vi "U8 Array Reverse Bit Order.vi"(1 "U8 Array Data In":u8[](array[numeric]) format="%02x") -> (0 "U8 Array Data Out":u8[](array[numeric]) format="%02x")   [LabVIEW 2016, in "SPIVI.lvlib"]
uses:
  SPIVI.lvlib
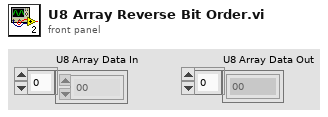
[diagram p1: front panel]
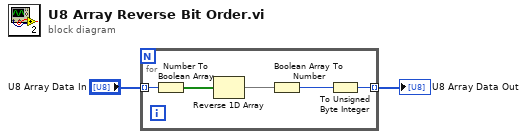
[diagram p0: block diagram]
diagram:
  n1 = for {
    tunnel: "U8 Array Data In" -> [w4] mode=indexing
    tunnel: [w3] -> w1 mode=indexing
    n2 = Number To Boolean Array(number=w4) -> (Boolean array=w7:bool[])
    n3 = Reverse 1D Array(array=w7) -> (reversed array=w6:bool[])
    n4 = Boolean Array To Number(Boolean array=w6) -> (number=w5:u32)
    n5 = To Unsigned Byte Integer(number=w5) -> (unsigned 8bit integer=w3:u8)
  }
  "U8 Array Data Out" <- w1
